vi "ParseVI.vi"(11 "vi ref":refnum<vi>) -> (2 "数组":string[][](array[string]), 3 "VIInfo":cluster{"Name":string, "Terminals":T1[]})   [LabVIEW 2018]
uses:
  Ctr/TerminalInfo.ctl
  Ctr/VIInfo.ctl
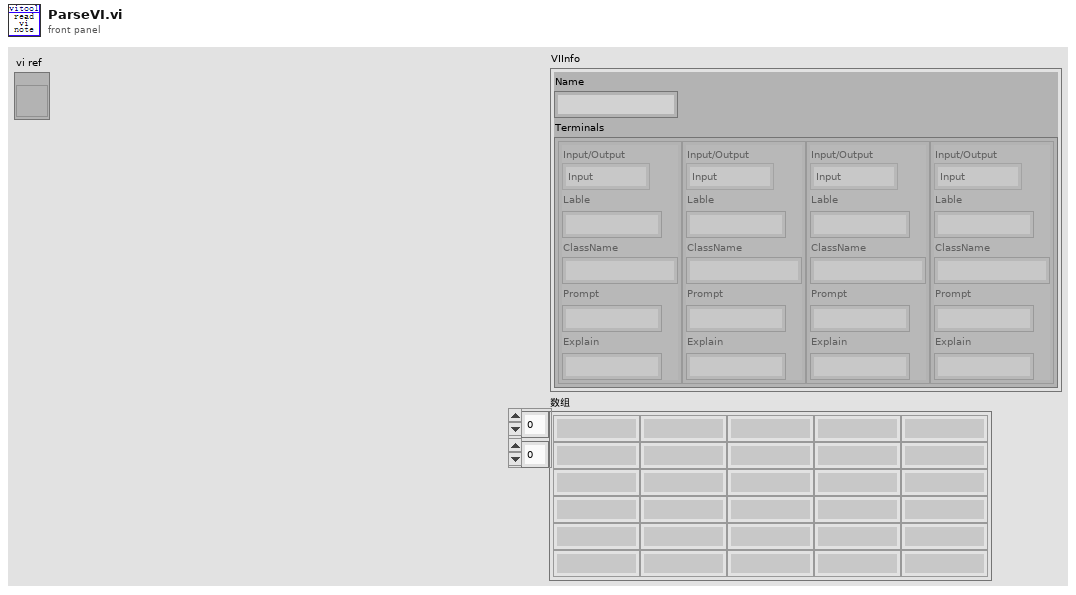
[diagram p1: front panel]
types:
  T1 = typedef "TerminalInfo.ctl" = cluster{"Input/Output":T2, "Lable":string, "ClassName":string, "Prompt":string, "Explain":string}
  T2 = typedef "IsIndicator" = enum16{"Input", "Output"}
  T3 = typedef "VIInfo.ctl" = cluster{"Name":string, "Terminals":T1[]}
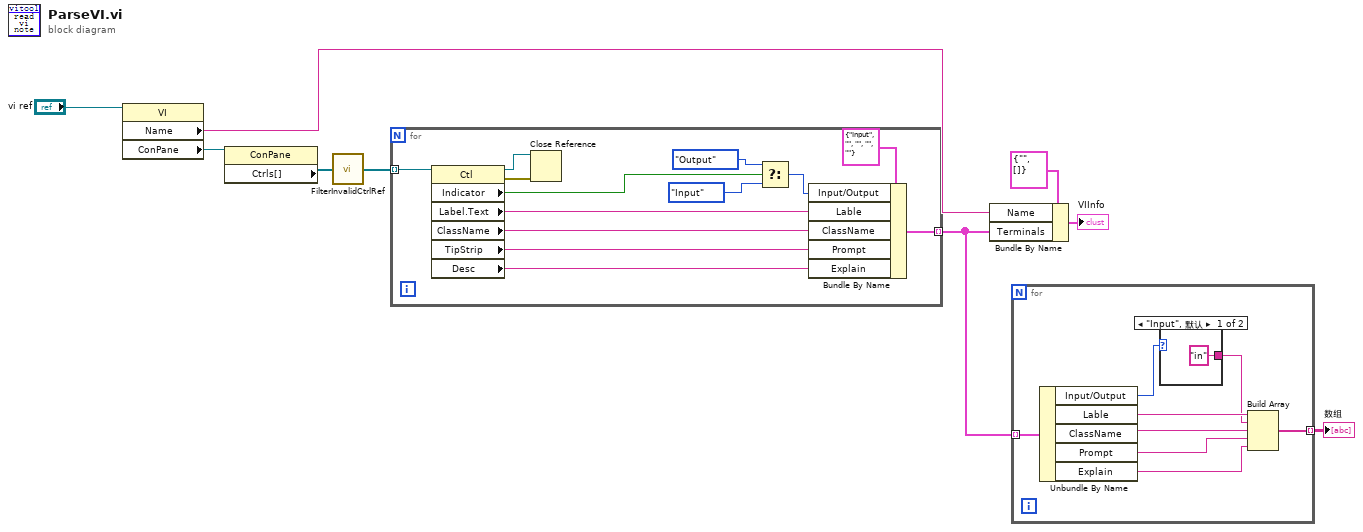
[diagram p0: block diagram]
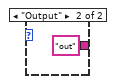
[diagram p2: hidden frame]
diagram:
  n1 = property class="VI"(reference="vi ref") -> ("Name"=w9:string, "ConPane"=w7:refnum<vi>)  [unwired: 1 in, 2 out]
  n2 = property class="ConPane"(reference=w7) -> ("Ctrls[]"=w5:refnum<vi>[])  [unwired: 1 in, 2 out]
  n3 = call "FilterInvalidCtrlRef.vi"("Ctrls in"=w5) -> ("Ctrl out"=w4:refnum<vi>[])
  n4 = for {
    tunnel: w4 -> [w22] mode=indexing
    tunnel: [w12] -> w3 mode=indexing
    n5 = property class="Ctl"(reference=w22) -> (reference out=w11:refnum<vi>, error out=w10:errorcluster, "Indicator"=w18:bool, "Label.Text"=w19:string, "ClassName"=w20:string, "TipStrip"=w14:string, "Desc"=w13:string)  [unwired: 1 in]
    n6 = Close Reference(reference=w11, error in (no error)=w10) -> ()  [unwired: 1 out]
    n7 = Select(t=IsIndicator."Output" ("Input/Output"), s=w18, f=IsIndicator."Input" ("Input/Output")) -> (s? t:f=w15:T2)
    n8 = Bundle By Name(cluster=T1 {"Input/Output"=enum."Input", "Lable"="", "ClassName"="", "Prompt"="", "Explain"=""} ("NewCluster"), "Input/Output"=w15, "Lable"=w19, "ClassName"=w20, "Prompt"=w14, "Explain"=w13) -> (w12:T1)
  }
  n9 = Bundle By Name(cluster=T3 {"Name"="", "Terminals"=[]} ("输入簇"), "Name"=w9, "Terminals"=w3) -> (→"VIInfo":T3)
  n10 = for {
    tunnel: w3 -> [w30] mode=indexing
    tunnel: [w23] -> w2 mode=indexing
    n11 = Unbundle By Name(w30) -> ("Input/Output"=w25:T2, "Lable"=w29:string, "ClassName"=w26:string, "Prompt"=w27:string, "Explain"=w28:string)
    n12 = case shown="\"Input\", 默认" w25 {
      tunnel: ["in" "out"] -> w24
      frame "Input", Default {
      }
      frame "Output" {
      }
    }
    n13 = Build Array(w29, w24, w26, w27, w28) -> (w23:string[])
  }
  "数组" <- w2
